vi "SendSET-NoListener.vi"(0 "connection ID":refnum<k5>, 1 "CommandArray":cluster{string[], u32[]}, 2 "ExpectedAnswer":string, 7 "Signature":u32, 11 "Error IN":errorcluster, 12 "Active SET":string, 13 "Value (little endianed byte array)":u8[](array[numeric])) -> (4 "connection ID (dup)":refnum<k5>, 8 "Succes":bool, 15 "Error OUT":errorcluster)   [LabVIEW 2011]
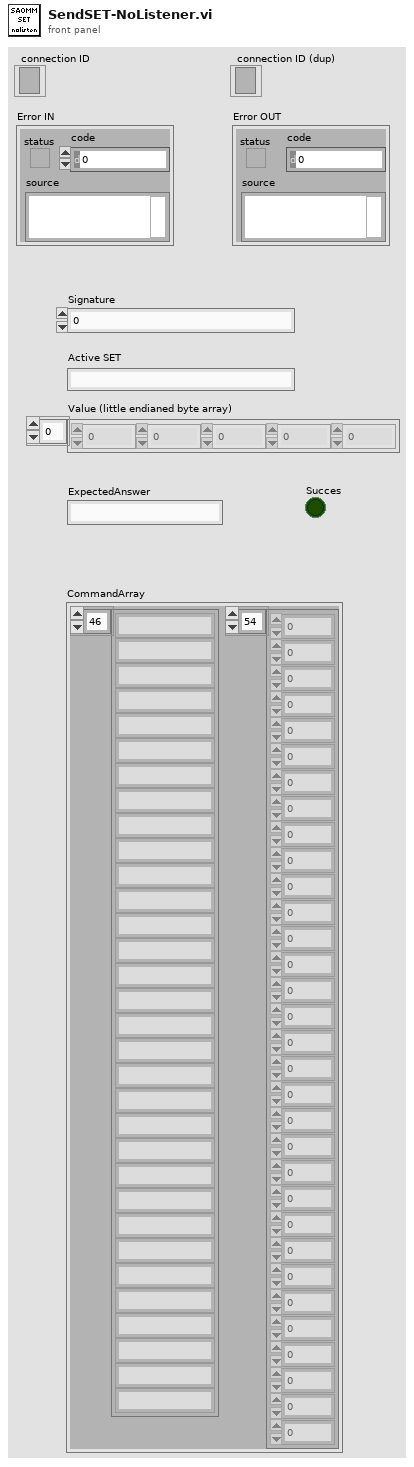
[diagram p1: front panel]
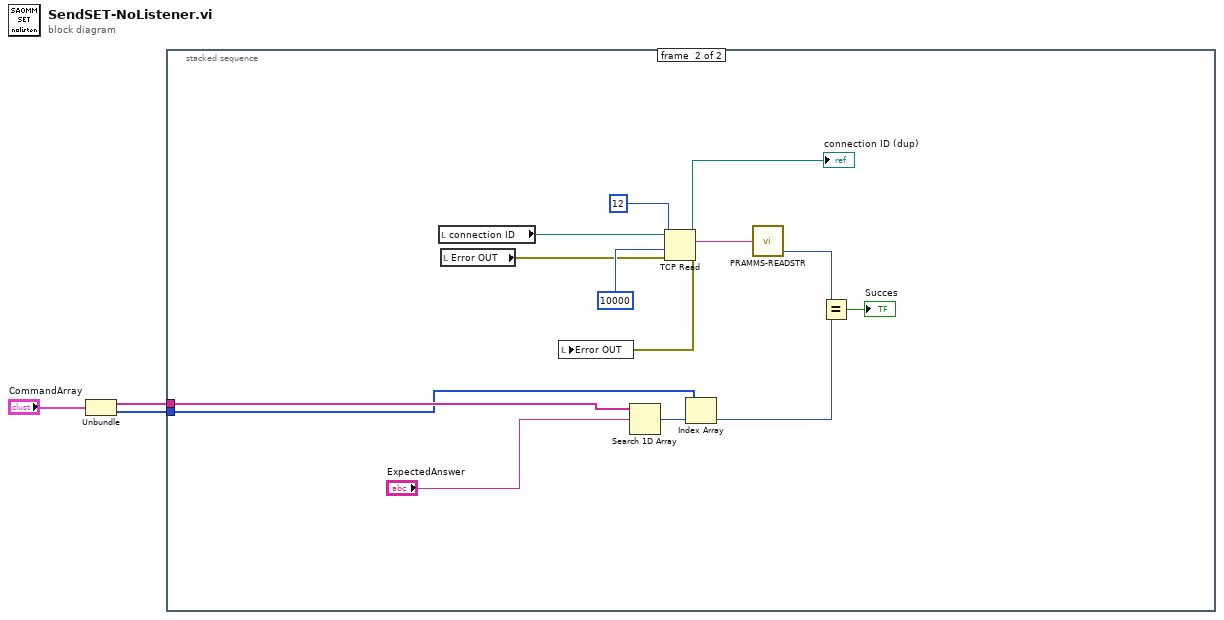
[diagram p0: block diagram]
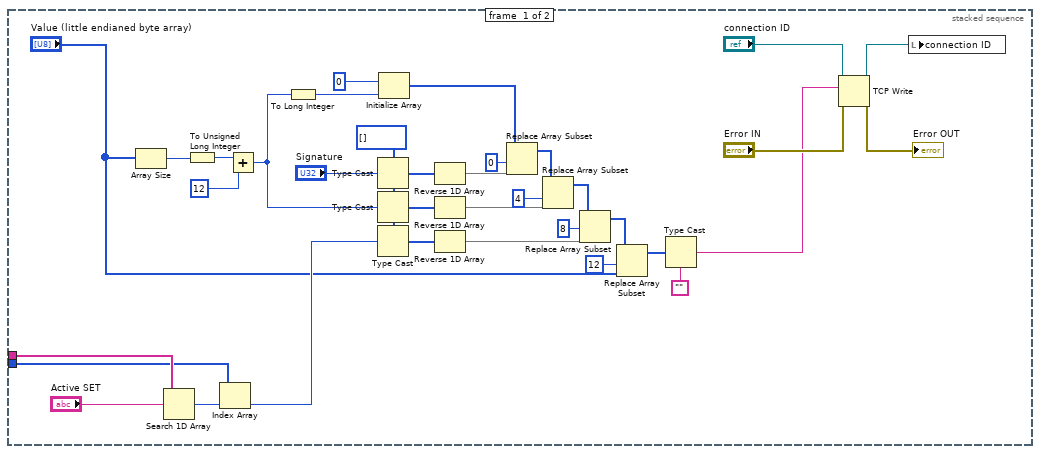
[diagram p2: hidden frame]
diagram:
  n1 = Unbundle("CommandArray") -> (w2:string[], w1:u32[])
  n2 = stacked-sequence {
    tunnel: w2 -> [w5 w40]
    tunnel: w1 -> [w4 w39]
    frame #0 {
      w37 = u8[] []
      n3 = Array Size(array="Value (little endianed byte array)") -> (size(s)=w38:i32)
      n4 = Search 1D Array(1D array=w5, element="Active SET") -> (index of element=w28:i32)  [unwired: 1 in]
      n5 = To Unsigned Long Integer(number=w38) -> (unsigned 32bit integer=w8:u32)
      n6 = Index Array(array=w4, index=w28) -> (element=w27:u32)
      n7 = Add(x=w8, y=u32 12 ("x")) -> (x+y=w25:u32)
      n8 = To Long Integer(number=w25) -> (32bit integer=w24:i32)
      n9 = Type Cast(type=w37, x="Signature") -> (*(type *) &x=w34:u8[])
      n10 = Type Cast(type=w37, x=w25) -> (*(type *) &x=w36:u8[])
      n11 = Type Cast(type=w37, x=w27) -> (*(type *) &x=w35:u8[])
      n12 = Initialize Array(u8 0, w24) -> (w16:u8[])
      n13 = Reverse 1D Array(array=w34) -> (reversed array=w12:u8[])
      n14 = Reverse 1D Array(array=w36) -> (reversed array=w11:u8[])
      n15 = Reverse 1D Array(array=w35) -> (reversed array=w10:u8[])
      n16 = Replace Array Subset(array=w16, new element=w12, index=0) -> (w23:u8[])
      n17 = Replace Array Subset(array=w23, new element=w11, index=4) -> (w22:u8[])
      n18 = Replace Array Subset(array=w22, new element=w10, index=8) -> (w21:u8[])
      n19 = Replace Array Subset(array=w21, new element="Value (little endianed byte array)", index=12) -> (w15:u8[])
      n20 = Type Cast(type="", x=w15) -> (*(type *) &x=w13:string)
      n21 = TCP Write(connection ID="connection ID", data in=w13, error in (no error)="Error IN") -> (connection ID out=w6:refnum<k5>, error out=→"Error OUT":errorcluster)  [unwired: 1 in, 1 out]
      n22 = local write "connection ID"(w6) -> ()
    }
    frame #1 {
      n23 = local read "connection ID"() -> (w48:refnum<k5>)
      n24 = local read "Error OUT"() -> (w47:errorcluster)
      n25 = Search 1D Array(1D array=w40, element="ExpectedAnswer") -> (index of element=w43:i32)  [unwired: 1 in]
      n26 = TCP Read(connection ID=w48, bytes to read=12, error in (no error)=w47, 9:10000 ("timeout ms (25000)")) -> (connection ID out=→"connection ID (dup)":refnum<k5>, data out=w51:string, error out=w46:errorcluster)  [unwired: 1 in]
      n27 = local write "Error OUT"(w46) -> ()
      n28 = Index Array(array=w39, index=w43) -> (element=w42:u32)
      n29 = call "PRAMMS-READSTR.vi"("String"=w51) -> ("Type"=w50:u32)  [unwired: 2 out]
      n30 = Equal?(x=w50, y=w42) -> (x = y?=→"Succes":bool)
    }
  }
